vi "Intake Height Handler.vi"(11 "JoystickDevRef":T1={"Device"=enum."USB 1"}) -> ()   [LabVIEW 2019]
uses:
  <vilib>/Rock Robotics/WPI/Joystick/WPI_JoystickDevRef.ctl
  <vilib>/Rock Robotics/WPI/Joystick/WPI_JoystickDeviceEnum.ctl
  Intake Operations.ctl
panel:
  in  "down scale":dbl
  in  "scale":dbl
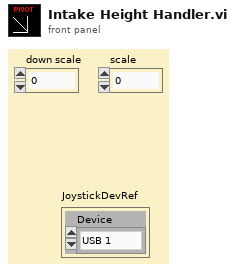
[diagram p1: front panel]
types:
  T1 = typedef "WPI_JoystickDevRef.ctl" = cluster{"Device":T2}
  T2 = typedef "WPI_JoystickDeviceEnum.ctl" = enum16{"USB 0", "USB 1", "USB 2", "USB 3", "USB 4", "USB 5"}
  T3 = typedef "Intake Operations.ctl" = enum16{"Reserve", "Read Current", "Immediate", "Immediate Height", "Intake Reserve"}
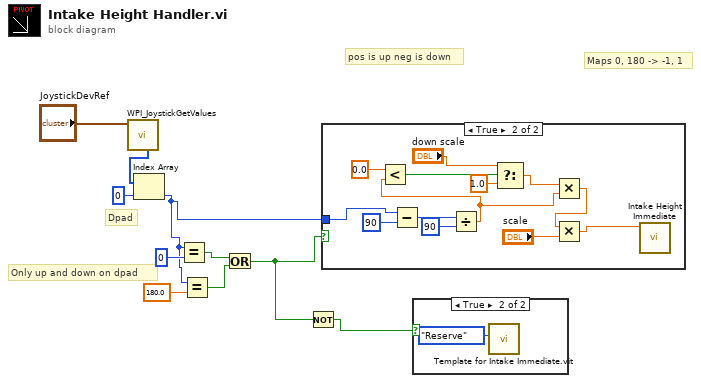
[diagram p0: block diagram]
diagram:
  # "Maps 0, 180 -> -1, 1"
  # "pos is up neg is down"
  # "Only up and down on dpad"
  # "Dpad"
  n1 = call <vilib>:"WPI_JoystickGetValues.vi"("JoystickDevRef"="JoystickDevRef") -> ("POVs"=w9:i16[])  [unwired: 6 in, 4 out]
  n2 = Index Array(array=w9, index=0) -> (element=w3:i16)
  n3 = Equal?(x=w3, y=i16 0) -> (x = y?=w5:bool)
  n4 = Equal?(x=w3, y=180.0) -> (x = y?=w4:bool)
  n5 = Or(x=w5, y=w4) -> (x .or. y?=w2:bool)
  n6 = Not(x=w2) -> (.not. x?=w1:bool)
  n7 = case shown="True" w2 {
    tunnel: w3 -> [_ w19]
    frame False {
    }
    frame True {
      n8 = Subtract(x=w19, y=i16 90) -> (x-y=w23:i16)
      n9 = Divide(x=w23, y=i16 90) -> (x/y=w13:dbl)
      n10 = Less?(x=0.0, y=w13) -> (x < y?=w17:bool)
      n11 = Select(t="down scale", s=w17, f=1.0) -> (s? t:f=w14:dbl)
      n12 = Multiply(x=w14, y=w13) -> (x*y=w12:dbl)
      n13 = Multiply(x=w12, y="scale") -> (x*y=w11:dbl)
      n14 = call "Intake Height Immediate.vi"("Setpoint"=w11) -> ()  [unwired: 10 in, 1 out]
    }
  }
  n15 = case shown="True" w1 {
    frame False {
    }
    frame True {
      n16 = call "Template for Intake Immediate.vit"("Operation"=Intake_Operations."Reserve") -> ()  [unwired: 10 in, 1 out]
    }
  }
